vi "fpga_integrator_AOD_framescan.vi"(8 "error in":errorcluster) -> (0 "error out":errorcluster)   [LabVIEW 2010]
uses:
  fpgaVIsAndControls/DDS_board_init_cluster.ctl
  fpgaVIsAndControls/FPGA_parameters_cluster.ctl
  common_typedefs/channels_cluster.ctl
  fpgaVIsAndControls/scan_points_cluster.ctl
  common_typedefs/gate_parameters_cluster.ctl
  <vilib>/Platform/TimedLoop/XDataNode/XDataNode.xnode
  <vilib>/Platform/TimedLoop/XDataNode/timing_clust.ctl
  <vilib>/Platform/TimedLoop/XDataNode/nitl_modes.ctl
  <vilib>/Platform/TimedLoop/XDataNode/wakeup.ctl
  common_typedefs/pixel_to_host_enum.ctl
  <vilib>/rvi/DataTransferAndStorage/Container/XNode/niFpgaContainer.xnode
  <vilib>/eio/EIONode/EIONode.xnode
  <vilib>/rvi/eio/nirviEIOImplementation/nirviEIOImplementation.xnode
  <vilib>/rvi/eio/common/nirviEmuClasses.ctl
  <vilib>/rvi/eio/nirviErrorMerge/nirviErrorMerge.xnode
  <vilib>/rvi/FIFO/Fifo_Resource/nirvififoEmulationSetSize.vi
  <vilib>/rvi/DataTransferAndStorage/Container/Common/niFpgaContainerGetUniqueNameForEmu.vi
  <vilib>/rvi/eio/common/nirviEmuTemplateMethod_noerrors.vi
  <vilib>/rvi/eio/common/nirviEmuTemplateMethod_errors.vi
  <vilib>/Platform/TimedLoop/XDataNode/XDNodeRunTimeDep.lvlib
panel:
  in  "gate 1":T1
  in  "gate 2":T1
  in  "gate 3":T1
  out "clock 2 state":bool
  out "clock 1 state":bool
  out "clock 3 state":bool
  out "acquiring?":bool
  in  "in triggered mode?":bool
  in  "stop at FIFO overflow?":bool
  in  "converter box version":i16=1 min=1 max=2
  out "scan points cluster out":T2
  in  "amplitude":u16=3400
  in  "y-point bandwidth":fxp<+,36,32>=10.0 format="%.28g"
  in  "x-point bandwidth":fxp<+,36,32>=10.0 format="%.28g"
  in  "amp comp":bool
  out "reset out":bool
  in  "inverse?":T3(ring)
  in  "OSK select":bool=TRUE
  in  "FPGA parameters in":T4 {"AOD center frequ. (Hz)_y" format="%.14g"; "AOD half bandwidth_y" format="%.14g"; "AOD Bandwidth_y (Hz)" format="%_6f"; "AOD center frequ. (Hz)_x" format="%.14g"; "cos Phi" format="%.35g"; "sin Phi" format="%.35g"; "AOD_Scale_Factor (1/Zoom)" format="%.35g"; "AOD half bandwidth_x" format="%.14g"; "AOD Bandwidth_x (Hz)" format="%_6f"}
  out "integrated pixel values":T5
  in  "maximum bit depth":i8=16
  in  "intergration iterations per pixel":u32=40
  in  "waiting iterations  per pixel":u32=200
  out "data read":T5
  in  "channel offsets":T5
  in  "number of pixels":i64=-1
  out "FIFO_DMA full?":bool
  out "current pixel no.":i64
  out "FPGA parameters out":T4 {"AOD center frequ. (Hz)_y" format="%.14g"; "AOD half bandwidth_y" format="%.14g"; "AOD Bandwidth_y (Hz)" format="%_6f"; "AOD center frequ. (Hz)_x" format="%.14g"; "cos Phi" format="%.35g"; "sin Phi" format="%.35g"; "AOD_Scale_Factor (1/Zoom)" format="%.35g"; "AOD half bandwidth_x" format="%.14g"; "AOD Bandwidth_x (Hz)" format="%_6f"}
  out "data sending counter (#bytes)":u32 caption="data sending counter"
  out "reset counter in":u8
  in  "acquire?":bool caption="Acquire?"
  in  "x-resolution":u16=10
  in  "y-resolution":u16=10
  in  "Stop complete VI":bool caption="Stop"
  in  "reset in":bool caption="Reset"
  in  "DDS board initialization parameters":T6={"Bypass PLL"=FALSE, "PLL Range"=TRUE, "Update Clock"=FALSE, "Triangle "=FALSE, "SDO Active"=FALSE, "LSB First"=FALSE, "OSK Int"=FALSE, "Output Shaped Keying Enable"=TRUE, "Bypass Sinc"=FALSE, "Digital Part"=TRUE, "OutPut DAC"=TRUE, "Control DAC"=FALSE, "Comparator"=FALSE, "Modus"=0, "Multiplier Value"=15} {"Modus" scale=0.0..4.0}
  # "IN"
  # "OUT"
  # "FPGA integrator"
  # "CONFIG"
  # "Clock parameters"
  # "DIO 1/32"
  # "PXI/RTSI 1"
  # "PXI/RTSI 2"
  # "FSK"
  # "Ramped"
  # "FSK"
  # "Chirp Modus"
  # "Unramped"
  # "BPSK"
  # "Single Tone"
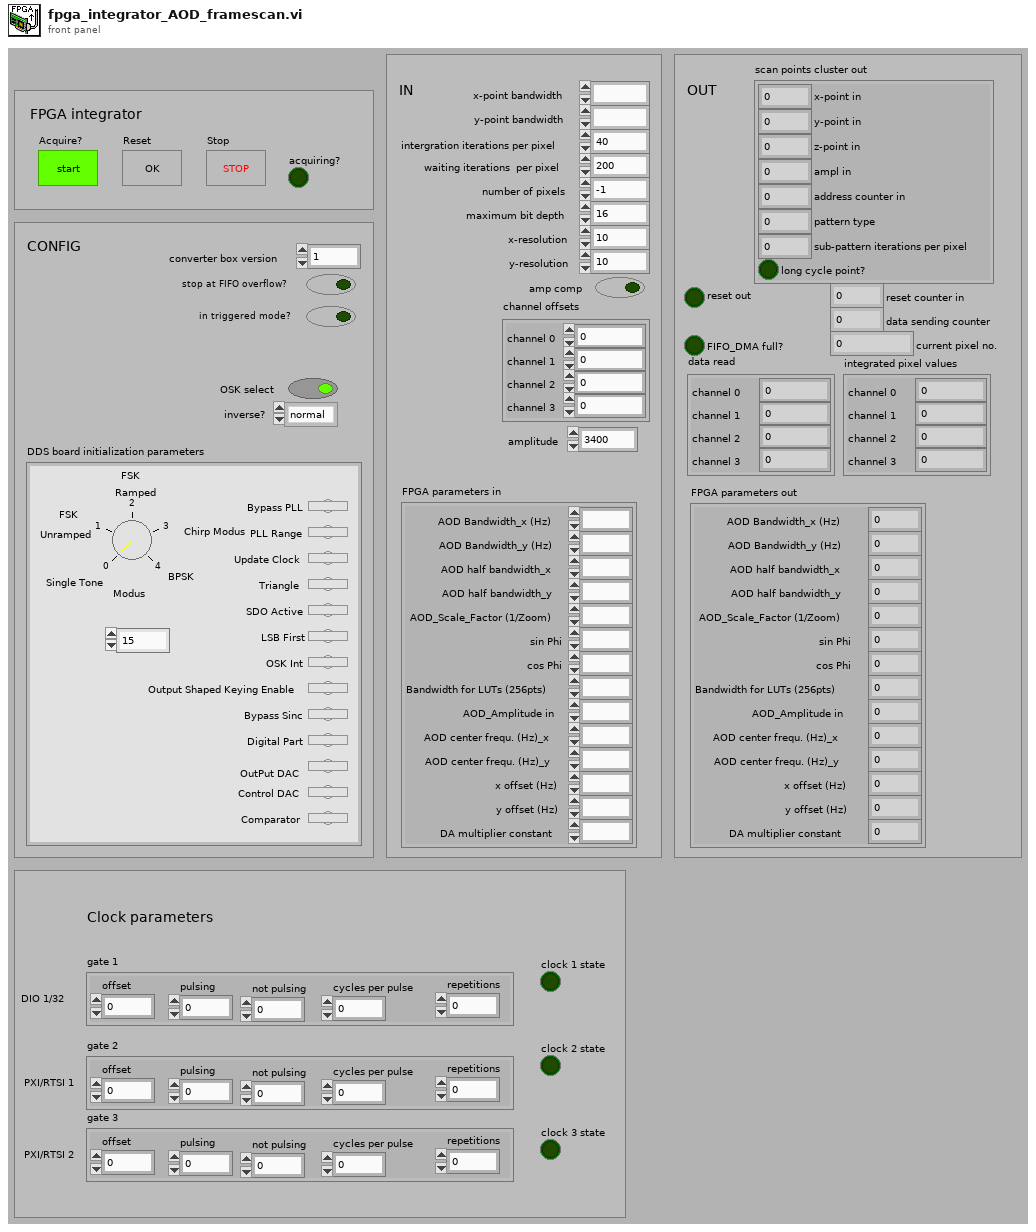
[diagram p1: front panel]
types:
  T1 = typedef "gate_parameters_cluster.ctl" = cluster{"offset":i64, "pulsing":i64, "not pulsing":i64, "cycles per pulse":i64, "repetitions":i64}
  T2 = typedef "scan_points_cluster.ctl" = cluster{"x-point in":u16, "y-point in":u16, "z-point in":u16, "ampl in":u16, "address counter in":i32, "pattern type":i8, "sub-pattern iterations per pixel":u16, "long cycle point?":bool}
  T3 = enum16{"normal", "x inversed", "y inversed", "x & y inversed"}
  T4 = typedef "FPGA_parameters_cluster.ctl" = cluster{"AOD Bandwidth_x (Hz)":fxp<+,36,32>, "AOD Bandwidth_y (Hz)":fxp<+,36,32>, "AOD half bandwidth_x":fxp<+,36,32>, "AOD half bandwidth_y":fxp<+,36,32>, "AOD_Scale_Factor (1/Zoom)":fxp<+,36,2>, "sin Phi":fxp<+/-,36,2>, "cos Phi":fxp<+/-,36,2>, "Bandwidth for LUTs (256pts)":fxp<+,36,0>, "AOD_Amplitude in":u16, "AOD center frequ. (Hz)_x":fxp<+,36,32>, "AOD center frequ. (Hz)_y":fxp<+,36,32>, "x offset (Hz)":fxp<+/-,36,32>, "y offset (Hz)":fxp<+/-,36,32>, "DA multiplier constant":fxp<+,64,4>}
  T5 = typedef "channels_cluster.ctl" = cluster{"channel 0":u32, "channel 1":u32, "channel 2":u32, "channel 3":u32}
  T6 = typedef "DDS_board_init_cluster.ctl" = cluster{"Bypass PLL":bool, "PLL Range":bool, "Update Clock":bool, "Triangle ":bool, "SDO Active":bool, "LSB First":bool, "OSK Int":bool, "Output Shaped Keying Enable":bool, "Bypass Sinc":bool, "Digital Part":bool, "OutPut DAC":bool, "Control DAC":bool, "Comparator":bool, "Modus":u8, "Multiplier Value":u8}
  T7 = typedef "FPGA_constants_cluster.ctl" = cluster{"register":cluster{"Reg. 1D":u8, "Reg. 1E":u8, "Reg. 1F":u8, "Reg. 20":u8}}
  T8 = typedef "XDNodeRunTimeDep.lvlib/timing_clust.ctl" = cluster{"Expected End [f-1]":u64, "Actual End [f-1]":u64, "Finished Late? [f-1]":bool, "Expected End [i-1]":u64, "Actual End [i-1]":u64, "Finished Late? [i-1]":bool, "Expected Start [i]":u64, "Actual Start [i]":u64, "Expected Start [f]":u64, "Actual Start [f]":u64, "Source Name":string, "Structure Name":string, "Period":i64, "Deadline":i64, "Offset":i64, "Start":i64, "Priority":i32, "Timeout":i32, "Mode":T9, "Wakeup Reason":T10, "Error":errorcluster, "Source Type":string, "Secondary Source Type":string, "Global End Time":u64, "Global Start Time":u64, "Frame Duration":u64, "Iteration Duration":u64, "Assigned CPU":i32, "I/O Scan Engine Mode":u32}
  T9 = typedef "XDNodeRunTimeDep.lvlib/nitl_modes.ctl" = enum32{"No Change", "Process missed periods, maintain original phase", "Discard missed periods, maintain original phase", "Process missed periods, ignore original phase", "Discard missed periods, ignore original phase"}
  T10 = typedef "XDNodeRunTimeDep.lvlib/wakeup.ctl" = enum32{"Normal", "Aborted", "Asynchronous wakeup", "Timing source error", "Timed loop error", "Timeout"}
  T11 = typedef "pixel_to_host_enum.ctl" = enum16{"3-channel mode", "4-channel mode"}
  T12 = typedef "DDS_board_values_cluster.ctl" = cluster{"y-frequency output":fxp<+,36,32>, "y-amplitude output":u16, "x-amplitude output":u16, "x-frequency output":fxp<+,36,32>, "z-position output":i16}
  T13 = typedef "nirviEmuClasses.ctl" = enum16{"IO Read", "IO Write", "Method", "Property Read", "Property Write"}
  T14 = typedef "gate_counters_cluster.ctl" = cluster{"phase iteration counter":i64, "phase repetition counter":i64, "pulse iteration counter":i64, "phase state":bool}
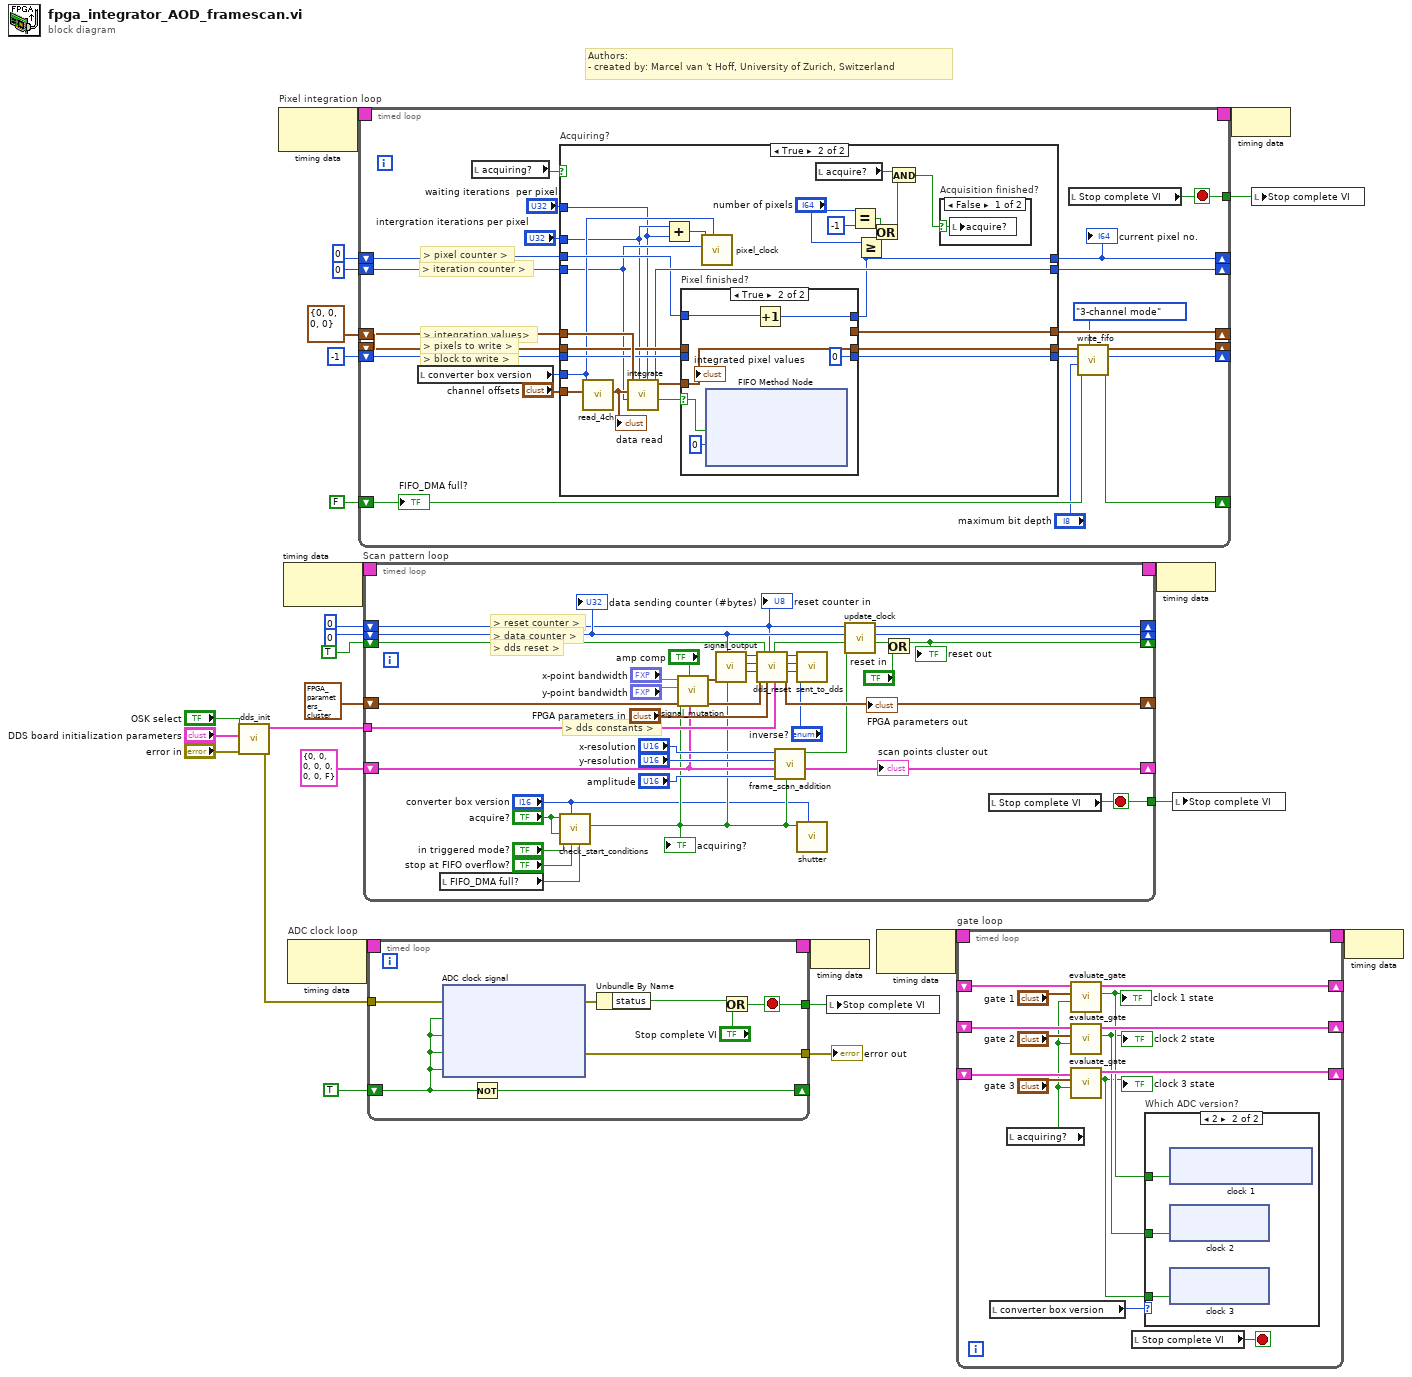
[diagram p0: block diagram]
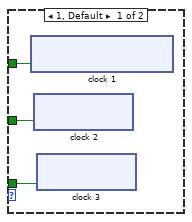
[diagram p2: hidden frame]
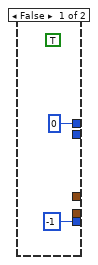
[diagram p3: hidden frame]
diagram:
  w8 = T5 {"channel 0"=0, "channel 1"=0, "channel 2"=0, "channel 3"=0} ("channel offsets 2")
  # "Authors: \n- created by: Marcel van 't Hoff, University of Zurich, Switzerland"
  n1 = call "dds_init.vi"("error in"="error in", "DDS board initialization parameters"="DDS board initialization parameters", "OSK select"="OSK select") -> ("error out"=w22:errorcluster, "constants out"=w23:T7)  [unwired: 7 in]
  n2 = node-c288() -> (w16:T8)  [unwired: 1 out]
  n3 = node-c288() -> (w10:T8)  [unwired: 1 in]
  n4 = node-c288() -> (w28:T8)  [unwired: 1 out]
  n5 = timed-loop "Pixel integration loop" {
    timing: w16 -> [_]
    timing-out: [_] -> w15
    shift-right: [w50] -> _
    shift-left: w8 -> [w49]
    shift-right: [w38] -> _
    shift-left: w8 -> [w48]
    shift-right: [w33] -> _
    shift-left: -1 ("block index out") -> [w47]
    shift-right: [w45] -> _
    shift-left: u32 0 ("iteration counter out") -> [w46]
    shift-right: [w43] -> _
    shift-left: i64 0 -> [w44]
    tunnel: [w42] -> w11
    shift-right: [w35] -> _
    shift-left: FALSE -> [w36]
    stop <- w42 stop-if-true
    # "> pixel counter >"
    # "> block to write >"
    # "> integration values>"
    # "> pixels to write >"
    # "> iteration counter >"
    n6 = local read "converter box version"() -> (w30:i16)
    n7 = local read "acquiring?"() -> (w29:bool)
    n8 = case "Acquiring?" shown="True" w29 {
      tunnel: [_ w74] -> w50
      tunnel: w49 -> [_ w77]
      tunnel: [_ w58] -> w37
      tunnel: w48 -> [_ w72]
      tunnel: w47 -> [_ w73]
      tunnel: w46 -> [_ w56]
      tunnel: [_ w71] -> w45
      tunnel: w44 -> [_ w62]
      tunnel: [i64 0 w61] -> w43
      tunnel: "channel offsets" -> [_ w60]
      tunnel: "intergration iterations per pixel" -> [_ w54]
      tunnel: "waiting iterations  per pixel" -> [_ w53]
      tunnel: [-1 ("block index out") w59] -> w34
      tunnel: w30 -> [_ w57]
      frame False {
        (unwired) TRUE
      }
      frame True {
        n9 = call "read_4ch.vi"("channel offsets"=w60, "converter box version"=w57) -> ("read output"=w75:T5)  [unwired: 9 in]
        "data read" <- w75
        n10 = call "integrate.vi"("waiting iterations per pixel"=w53, "integration iterations per pixel"=w54, "iteration counter in"=w56, "sampling values in"=w75, "previous pixel values in"=w77) -> ("finished?"=w64:bool, "iteration counter out"=w71:u32, "new pixel values out"=w76:T5)  [unwired: 4 in]
        n11 = Add(x=w54, y=w53) -> (x+y=w55:u32)
        n12 = case "Pixel finished?" shown="True" w64 {
          selector: w64 -> [_ w87]
          tunnel: w76 -> [w82 w88]
          tunnel: [w82 _] -> w74
          tunnel: w73 -> [w81 _]
          tunnel: [w81 0 ("block index out")] -> w59
          tunnel: w72 -> [w80 _]
          tunnel: [w80 w88] -> w58
          tunnel: w62 -> [w79 w85]
          tunnel: [w79 w84] -> w61
          frame False {
          }
          frame True {
            n13 = xnode ("FIFO Method Node")("Element"=w87, "Timeout"=0) -> ()  [unwired: 1 in, 2 out]
            n14 = Increment(x=w85) -> (x+1=w84:i64)
            "integrated pixel values" <- w88
          }
        }
        n15 = call "pixel_clock.vi"("converter box version"=w57, "current iteration"=w56, "iterations per pixel"=w55) -> ()  [unwired: 9 in]
        n16 = local read "acquire?"() -> (w69:bool)
        n17 = Equal?(x="number of pixels", y=i64 -1 ("x")) -> (x = y?=w67:bool)
        n18 = Greater Or Equal?(x="number of pixels", y=w61) -> (x >= y?=w66:bool)
        n19 = Or(x=w67, y=w66) -> (x .or. y?=w68:bool)
        n20 = And(x=w69, y=w68) -> (x .and. y?=w70:bool)
        n21 = case "Acquisition finished?" shown="False" w70 {
          selector: w70 -> [w78 _]
          frame False {
            n22 = local write "acquire?"(w78) -> ()
          }
          frame True {
          }
        }
      }
    }
    "current pixel no." <- w43
    n23 = local read "Stop complete VI"() -> (w42:bool)
    n24 = call "write_fifo.vi"("pixel-to-host\n mode"=pixel_to_host_enum."3-channel mode" ("pixel-to-host\n mode"), "FIFO overflow in"=w36, "maximum bit depth"="maximum bit depth", "block index in"=w34, "values to be written"=w37) -> ("FIFO overflow out"=w35:bool, "block index out"=w33:i32, "channels out"=w38:T5)  [unwired: 4 in]
    "FIFO_DMA full?" <- w36
  }
  n25 = timed-loop "Scan pattern loop" {
    tunnel: [w173] -> w24
    tunnel: w23 -> [w163]
    shift-right: [w160] -> _
    shift-left: T4 {"AOD Bandwidth_x (Hz)"=35000000.0, "AOD Bandwidth_y (Hz)"=35000000.0, "AOD half bandwidth_x"=17500000.0, "AOD half bandwidth_y"=17500000.0, "AOD_Scale_Factor (1/Zoom)"=0.0, "sin Phi"=0.0, "cos Phi"=1.0, "Bandwidth for LUTs (256pts)"=0.0, "AOD_Amplitude in"=1, "AOD center frequ. (Hz)_x"=0.0, "AOD center frequ. (Hz)_y"=3400.0, "x offset (Hz)"=94000000.0, "y offset (Hz)"=94000000.0, "DA multiplier constant"=0.0} ("FPGA parameters out 2") -> [w153]
    shift-right: [w170] -> _
    shift-left: TRUE ("reset dds out") -> [w155]
    shift-right: [w168] -> _
    shift-left: u32 0 ("data sending counter (#bytes)") -> [w167]
    shift-right: [w166] -> _
    shift-left: u8 0 ("reset counter in") -> [w162]
    timing: w10 -> [_]
    timing-out: [_] -> w9
    shift-right: [w150] -> _
    shift-left: T2 {"x-point in"=0, "y-point in"=0, "z-point in"=0, "ampl in"=0, "address counter in"=0, "pattern type"=0, "sub-pattern iterations per pixel"=0, "long cycle point?"=FALSE} ("scan points cluster out") -> [w149]
    stop <- w173 stop-if-true
    # "> dds constants >"
    # "> data counter >"
    # "> reset counter >"
    # "> dds reset >"
    n26 = local read "FIFO_DMA full?"() -> (w146:bool)
    n27 = call "check_start_conditions.vi"("FIFO overflow?"=w146, "stop at FIFO overflow?"="stop at FIFO overflow?", "converter box version"="converter box version", "already acquiring?"="acquire?", "in triggered mode?"="in triggered mode?", "acquire"="acquire?") -> ("acquire?"=w143:bool)  [unwired: 5 in]
    "acquiring?" <- w143
    n28 = call "signal_mutation.vi"("scan points cluster in"=w149, "amplitude compensation?"="amp comp", "FPGA parameters in"=w153, "acquire?"=w143, "y point bandwidth"="y-point bandwidth", "x point bandwidth"="x-point bandwidth") -> ("FPGA parameters out"=w156:T4, "cluster out"=w169:T12)  [unwired: 4 in]
    n29 = call "signal_output.vi"("acquire?"=w143, "pipeline counter in"=w167, "cluster in"=w169) -> ("address bits out"=w177:u8, "y data bits out"=w178:u8, "x data bits out"=w179:u8)  [unwired: 6 in]
    n30 = call "dds_reset.vi"("DDS data bits in"=w179, "DDS0 data bits in"=w178, "address bits in"=w177, "FPGA parameters in"=w156, "reset dds in"=w155, "counter in"=w162, "FPGA parameters reset"="FPGA parameters in", "constants in"=w163) -> ("reset dds out"=w165:bool, "DDS0 data bits out"=w176:u8, "DDS1 data bits out"=w175:u8, "address bits out"=w174:u8, "FPGA parameters out"=w160:T4)  [unwired: 7 in]
    "FPGA parameters out" <- w160
    n31 = call "frame_scan_addition.vi"("frame scanning?"=w143, "amplitude"="amplitude", "scan points cluster in"=w149, "y-resolution"="y-resolution", "x-resolution"="x-resolution") -> ("scan points cluster out"=w150:T2, "new pixel update?"=w157:bool)  [unwired: 5 in]
    "scan points cluster out" <- w150
    n32 = call "sent_to_dds.vi"("inversion selector"="inverse?", "address bits in"=w174, "DDS1 input"=w175, "DDS0 input"=w176) -> ()  [unwired: 8 in]
    n33 = call "shutter.vi"("converter box version"="converter box version", "open?"=w143) -> ()  [unwired: 10 in]
    n34 = call "update_clock.vi"("update command in"=w157, "update reset counter in"=w165, "data sending counter (#bytes) in"=w167, "reset counter in"=w162) -> ("update reset counter out"=w161:bool, "data sending counter (#bytes) out"=w168:u32, "reset counter out"=w166:u8)  [unwired: 5 in]
    n35 = Or(x=w161, y="reset in") -> (x .or. y?=w170:bool)
    "reset out" <- w170
    n36 = local read "Stop complete VI"() -> (w173:bool)
    "reset counter in" <- w162
    "data sending counter (#bytes)" <- w167
  }
  n37 = timed-loop "ADC clock loop" {
    timing: w28 -> [_]
    timing-out: [_] -> w27
    shift-right: [w183] -> _
    shift-left: TRUE -> [w188]
    tunnel: [w185] -> w25
    tunnel: w22 -> [w184]
    tunnel: [w182] -> w7
    stop <- w185 stop-if-true
    n38 = xnode "ADC clock signal"("error in"=w184, "Connector0/DIO14"=w188, "Connector0/DIO15"=w188, "Connector1/DIO14"=w188, "Connector1/DIO15"=w188) -> ("error out"=w182:errorcluster)  [unwired: 4 in, 4 out]
    n39 = Not(x=w188) -> (.not. x?=w183:bool)
    n40 = Unbundle By Name(w182) -> ("status"=w186:bool)
    n41 = Or(x=w186, y="Stop complete VI") -> (x .or. y?=w185:bool)
  }
  "error out" <- w7
  n42 = node-c288(w27) -> ()
  n43 = local write "Stop complete VI"(w25) -> ()
  n44 = node-c288() -> (w2:T8)  [unwired: 1 in]
  n45 = timed-loop "gate loop" {
    timing: w2 -> [_]
    timing-out: [_] -> w1
    shift-right: [w299] -> _
    shift-left: _ -> [w300]
    shift-right: [w297] -> _
    shift-left: _ -> [w298]
    shift-right: [w296] -> _
    shift-left: _ -> [w295]
    stop <- w287 stop-if-true
    n46 = local read "converter box version"() -> (w288:i16)
    n47 = local read "acquiring?"() -> (w286:bool)
    n48 = call "evaluate_gate.vi"("acquiring?"=w286, "gate settings"="gate 1", "gate counters in"=w300) -> ("pulse state out"=w291:bool, "gate counters out"=w299:T14)  [unwired: 7 in]
    "clock 1 state" <- w291
    n49 = call "evaluate_gate.vi"("acquiring?"=w286, "gate settings"="gate 2", "gate counters in"=w298) -> ("pulse state out"=w290:bool, "gate counters out"=w297:T14)  [unwired: 7 in]
    "clock 2 state" <- w290
    n50 = call "evaluate_gate.vi"("acquiring?"=w286, "gate settings"="gate 3", "gate counters in"=w295) -> ("pulse state out"=w289:bool, "gate counters out"=w296:T14)  [unwired: 7 in]
    "clock 3 state" <- w289
    n51 = local read "Stop complete VI"() -> (w287:bool)
    n52 = case "Which ADC version?" shown="2" w288 {
      tunnel: w291 -> [w301 w339]
      tunnel: w290 -> [w302 w338]
      tunnel: w289 -> [w303 w337]
      frame 1, Default {
        n53 = xnode "clock 1"("Connector1/DIO32"=w301) -> ()  [unwired: 1 in, 1 out]
        n54 = xnode "clock 2"("PXI_RTSI_1"=w302) -> ()  [unwired: 1 in, 1 out]
        n55 = xnode "clock 3"("PXI_RTSI_2"=w303) -> ()  [unwired: 1 in, 1 out]
      }
      frame 2 {
        n56 = xnode "clock 1"("Connector0/DIO38"=w339) -> ()  [unwired: 1 in, 1 out]
        n57 = xnode "clock 2"("PXI_RTSI_1"=w338) -> ()  [unwired: 1 in, 1 out]
        n58 = xnode "clock 3"("PXI_RTSI_2"=w337) -> ()  [unwired: 1 in, 1 out]
      }
    }
  }
  n59 = node-c288(w9) -> ()
  n60 = local write "Stop complete VI"(w24) -> ()
  n61 = node-c288(w15) -> ()
  n62 = local write "Stop complete VI"(w11) -> ()
  n63 = node-c288(w1) -> ()
